vi "midterm_3.vi"() -> ()   [LabVIEW 2024]
uses:
  <userlib>/ME121-25-main/ME121-25-main/LabVIEW/SerialVIs/subs/portX.xctl
panel:
  in  "stop 3":bool
  out "Starting postion":cluster{"X":i32, "Y":i32}
  out "Ending Position":cluster{"X":i32, "Y":i32}
  out "2D Picture":picture
  in  "stop":bool
  in  "Initial Postion":cluster{"x-position":dbl, "y-position":dbl} {"y-position" scale=0.0..162.5; "x-position" scale=0.0..162.5}
  in  "Final Position":cluster{"x-position":dbl, "y-position":dbl} {"y-position" scale=0.0..162.5; "x-position" scale=0.0..162.5}
  out "Arms":picture
  in  "portX 2":refnum<visa-resource-name>(xcontrol)="ASRL15"
  in  "end effector":cluster{dbl, dbl}={159.01647214211073, 1.9100783062530127} {"?" format="%.1f"; "?" format="%#.1f"}
  in  "L 2":dbl(slide)=85.0 scale=0.0..200.0
  in  "L 1":dbl(slide)=77.5 scale=0.0..200.0
  out "resulting string":string="move(-43,72, -29)"
  # "Advance Dynamics - Midterm - 3DoF Arm"
  # "VI Overview\n\nThis LabVIEW VI controls a 3DoF robotic arm with two links and a chair attached to the end effector. \nThe objective is to move the arm while keeping the chair level to prevent a seated LEGO figure from falling.\nFeatures:\n\n    - Select initial and final positions\n    - Perform inverse kinematics (IK) to compute joint angles\n    - Communicate with a microcontroller to send movement commands\n    - Display a 2D visualization of the arm and its reachable workspace"
  # "1 - Select Port"
  # "User Guide:\n\n    1- Connect to the microcontroller via the port on the right.\n    2 -Select initial and final positions.\n    3 - Click Run:\n       - If the position is within range, a 2D visualization appears, and the user is prompted to execute the                                            \n          movement.\n       -  If out of range, the user is asked to select a valid position.\n\nLet me know if you need further refinements!"
  # "Set an initial position"
  # "mm"
  # "mm"
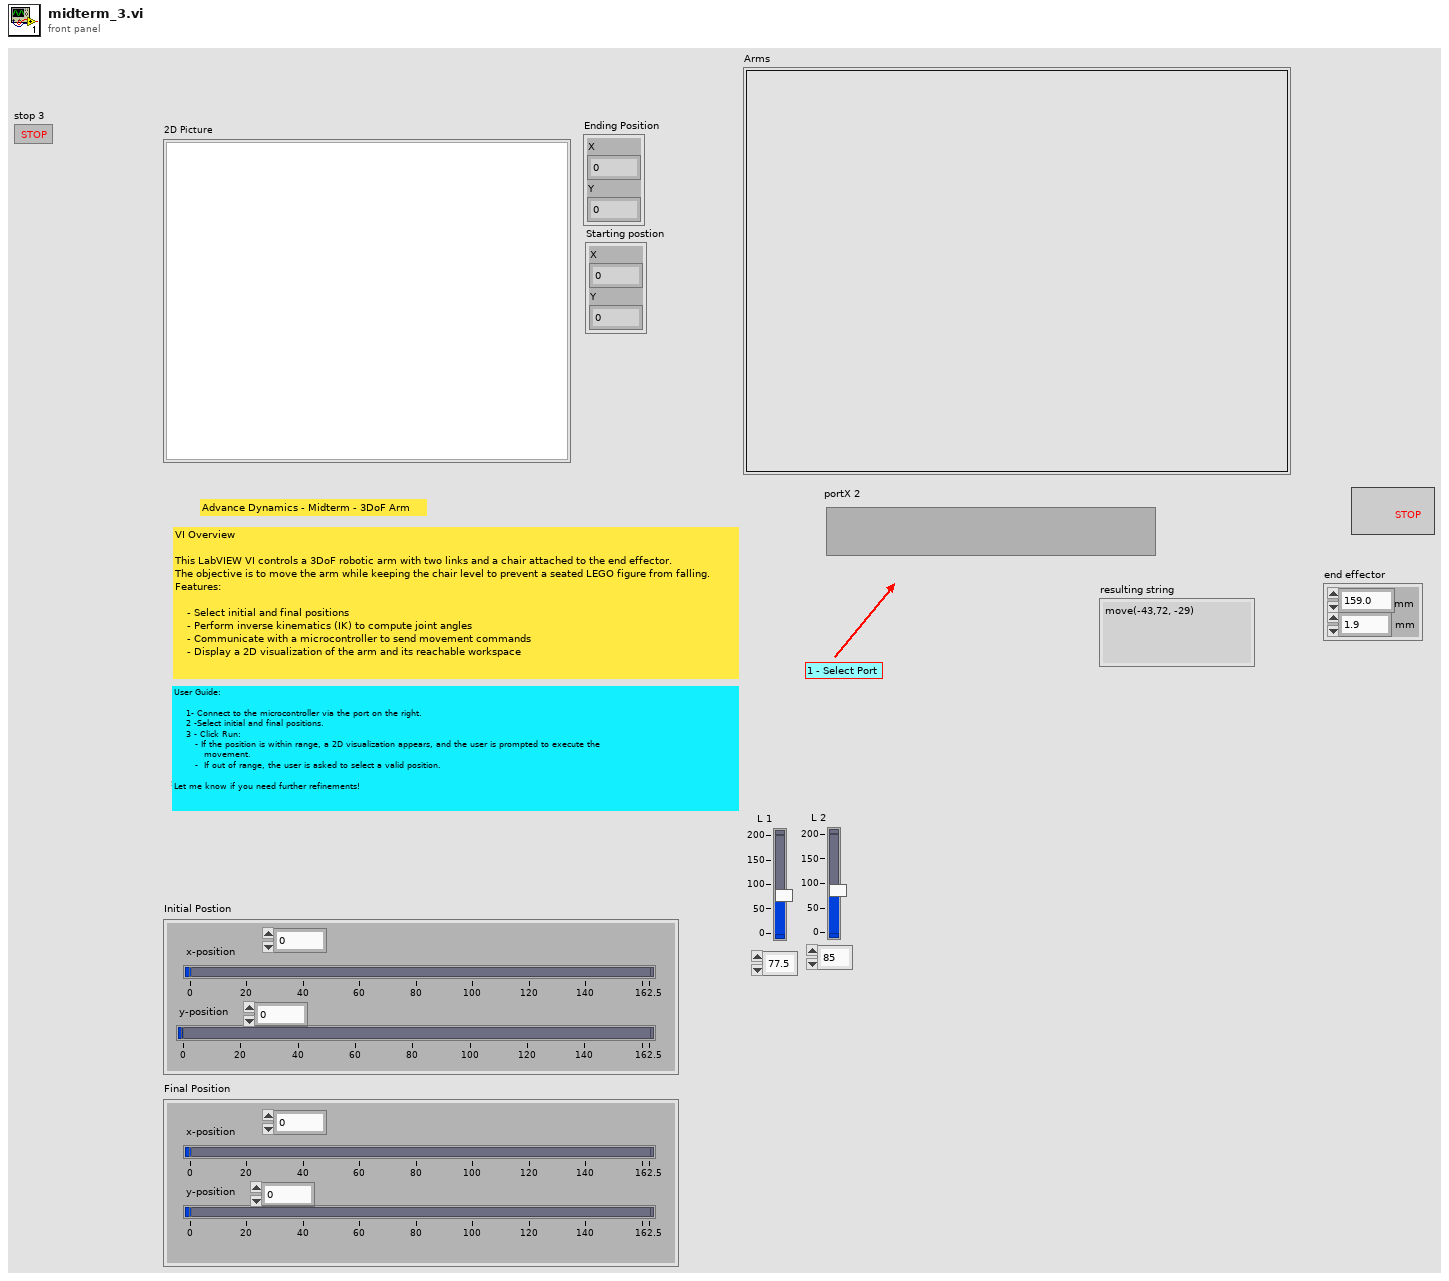
[diagram p1: front panel]
types:
  T1 = cluster{"Width":u16, "Style":enum32{"Solid", "Dash", "Dot", "DashDot", "DashDotDot"}}
  T2 = typedef "lveventtype.ctl" = enum32{"Null", "Timeout", "Annotation Menu Selection", "Annotation Menu Selection?", "App Instance Close", "App Instance Close?", "Autoscale Range Change", "Bookmark Info Change", "Cell Edit", "Cell Edit?", "Cursor Grab", "Cursor Grab?", "Cursor Menu Selection", "Cursor Menu Selection?", "Cursor Move", "Cursor Release", "Data Change", "Direction Change", "Display State Change", "Drag Ended", "Drag Enter", "Drag Leave", "Drag Over", "Drag Source Update", "Drag Starting", "Drag Starting?", "Drop", "Exec State Change", "Key Down", "Key Down?", "Key Repeat", "Key Repeat?", "Key Up", "Listbox Double Click", "Menu Activation?", "Menu Selection (App)", "Menu Selection? (App)", "Menu Selection (User)", "Mouse Down", "Mouse Down?", "Mouse Enter", "Mouse Leave", "Mouse Move", "Mouse Up", "Mouse Wheel", "NI Security User Change (App)", "Pane Size", "Panel Close", "Panel Close?", "Panel Resize", "Plot Attribute Change", "Scale Range Change", "Shortcut Menu Activation?", "Shortcut Menu Selection (App)", "Shortcut Menu Selection? (App)", "Shortcut Menu Selection (User)", "Tree Double Click", "Tree Drag", "Tree Drag?", "Tree Drop", "Tree Drop?", "Tree Item Close", "Tree Item Close?", "Tree Item Open", "Tree Item Open?", "User Event", "Value Change"}
  T3 = typedef "LVMouseTypeDef.ctl" = cluster{"Mouse Position":cluster{"X":i32, "Y":i32}, "Mouse Modifiers":cluster{"Button Down":bool, "Shift Mod":bool, "Menu Mod":bool, "Option Mod":bool}}
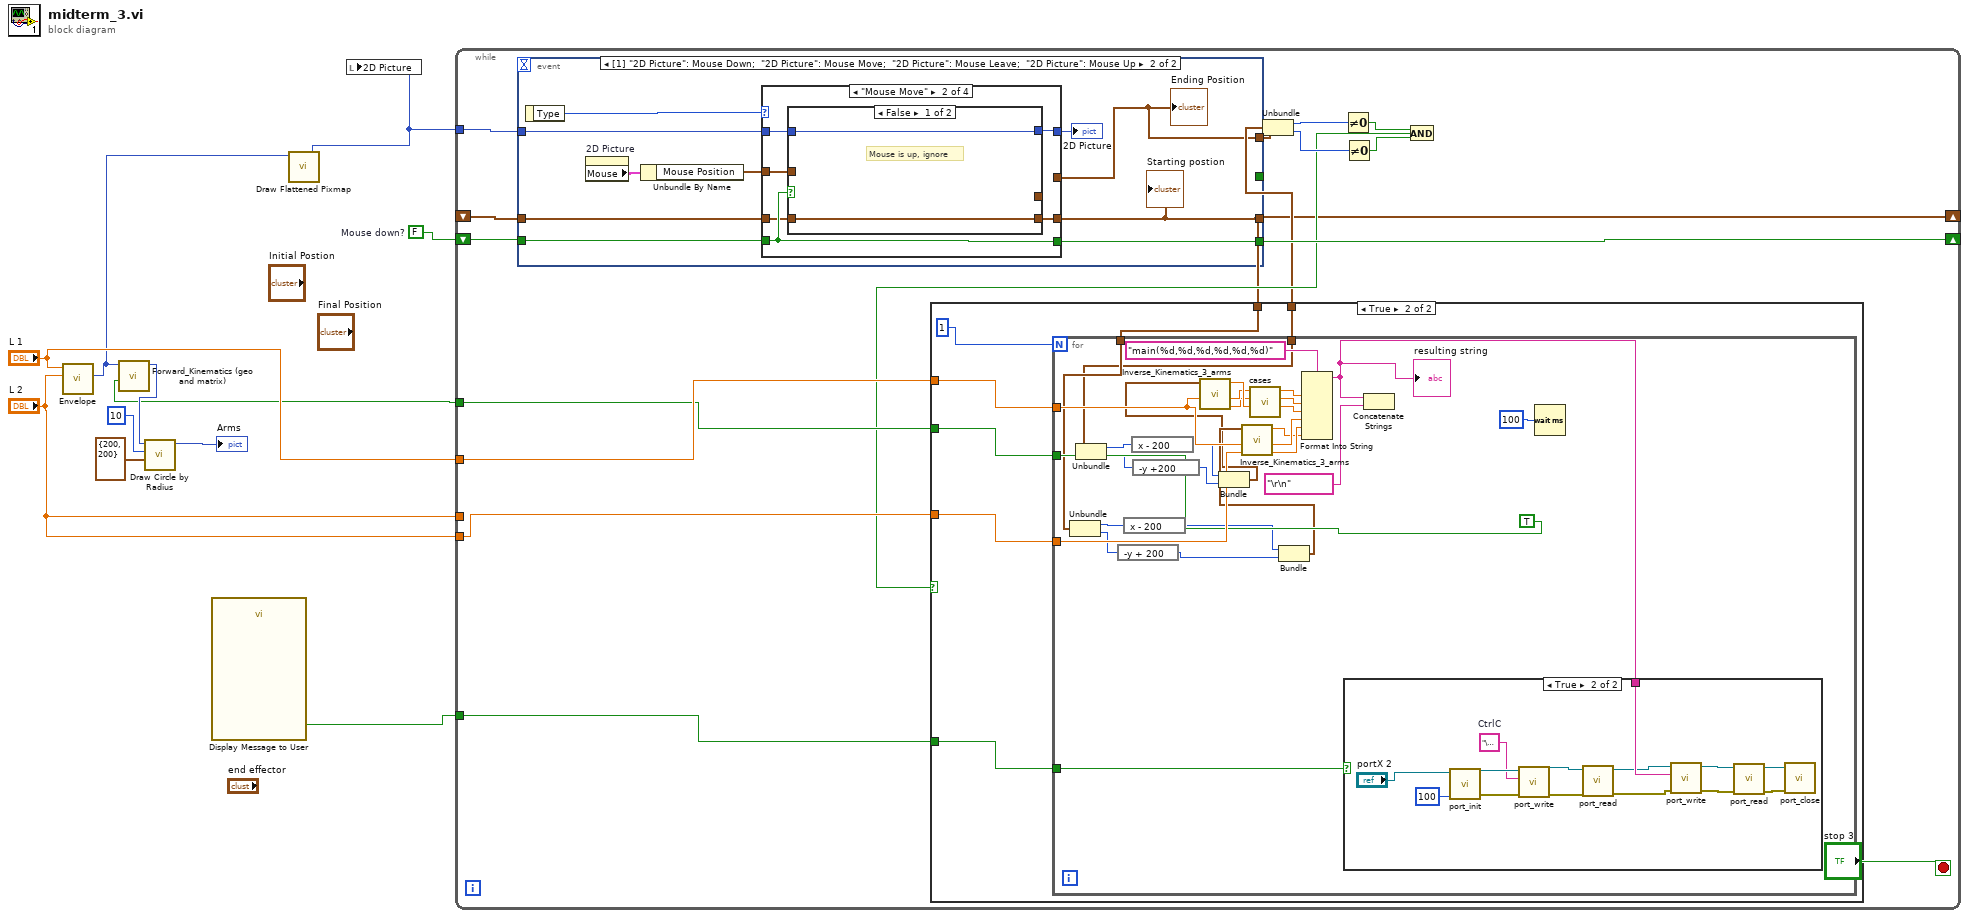
[diagram p0: block diagram]
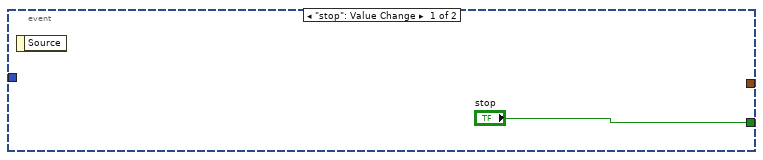
[diagram p4: hidden frame]
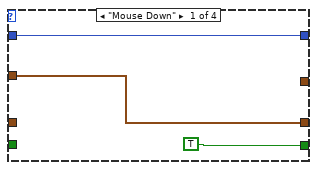
[diagram p5: hidden frame]
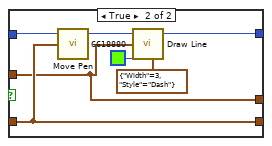
[diagram p6: hidden frame]
diagram:
  w10 = FALSE  # Mouse down?
  n1 = call "Envelope.vi"("L 2"="L 2", "L 1"="L 1") -> ("new picture"=w1:picture)  [unwired: 9 in]
  n2 = call "Display Message to User"() -> ("OK"=w2:bool)  [unwired: 10 in, 1 out]
  n3 = call <vilib>:"Draw Flattened Pixmap.vi"("picture"=w1) -> ("new picture"=w11:picture)  [unwired: 8 in]
  n4 = local write "2D Picture"(w11) -> ()
  n5 = while {
    tunnel: w11 -> [w27]
    shift-right: [w26] -> _
    shift-left: w10 -> [w25]
    shift-right: [w12] -> _
    shift-left: _ -> [w24]
    tunnel: "L 1" -> [w23]
    tunnel: "L 2" -> [_]
    tunnel: "L 2" -> [w22]
    tunnel: [w21] -> w3
    tunnel: w2 -> [w20]
    stop <- "stop 3" stop-if-true
    n6 = event shown="[1] \"2D Picture\": Mouse Down;  \"2D Picture\": Mouse Move;  \"2D Picture\": Mouse Leave;  \"2D Picture\": Mouse Up" {
      selector: _ -> [_ _]
      dyn-events: _ -> [_ _]
      timeout: _ -> [_ _]
      tunnel: ["stop" _] -> _
      tunnel: w27 -> [_ w86]
      tunnel: [_ w88] -> w26
      tunnel: w25 -> [_ w83]
      tunnel: [_ w82] -> w12
      tunnel: w24 -> [_ w81]
      tunnel: [_ w79] -> w13
      event "stop": Value Change {
        n7 = event-data() -> ()  [unwired: 1 in, 1 out]
      }
      event "2D Picture": Mouse Down; "2D Picture": Mouse Move; "2D Picture": Mouse Leave; "2D Picture": Mouse Up {
        n8 = event-data() -> ("Type"=w87:T2)  [unwired: 1 in]
        n9 = property on="2D Picture" class="Pict"() -> ("Mouse"=w84:T3)  [unwired: 2 in, 2 out]
        n10 = Unbundle By Name(w84) -> ("Mouse Position"=w80:cluster{"X":i32, "Y":i32})
        n11 = case shown="\"Mouse Move\"" w87 {
          tunnel: [TRUE ("fill?(F)") w94 _ _] -> w88
          tunnel: w86 -> [w89 w96 w108 w109]
          tunnel: [w89 w97 w108 w109] -> w85
          tunnel: w80 -> [w90 w95 _ w111]
          tunnel: w83 -> [_ w94 _ _]
          tunnel: [w90 w93 w107 w110] -> w82
          tunnel: w81 -> [_ w92 w107 w110]
          tunnel: [_ _ _ w111] -> w79
          frame "Mouse Down" {
          }
          frame "Mouse Move" {
            n12 = case shown="False" w94 {
              tunnel: [w99 w106] -> w97
              tunnel: w96 -> [w99 w104]
              tunnel: w95 -> [_ w100]
              tunnel: [w98 w102] -> w93
              tunnel: w92 -> [w98 w102]
              tunnel: [_ w100] -> _
              frame False {
                # "Mouse is up, ignore"
              }
              frame True {
                n13 = call <vilib>:"Move Pen.vi"("new position"=w102, "picture"=w104) -> ("new picture"=w103:picture)  [unwired: 3 in]
                n14 = call <vilib>:"Draw Line.vi"("picture"=w103, "end point"=w100, "color(black)"=u32 6618880, "pen"=T1 {"Width"=3, "Style"=enum."Dash"}) -> ("new picture"=w106:picture)  [unwired: 5 in]
              }
            }
          }
          frame Default {
            # "reset on mouse up, mouse leave, etc."
          }
          frame "Mouse Up" {
          }
        }
        "2D Picture" <- w85
        "Ending Position" <- w79
        "Starting postion" <- w82
      }
    }
    n15 = Unbundle(w13) -> ("X"=w18:i32, "Y"=w17:i32)
    n16 = Not Equal To 0?(x=w18) -> (x != 0?=w15:bool)
    n17 = Not Equal To 0?(x=w17) -> (x != 0?=w16:bool)
    n18 = And(x=w15, y=w16) -> (x .and. y?=w14:bool)
    n19 = case shown="True" w14 {
      tunnel: w23 -> [_ w33]
      tunnel: w22 -> [_ w32]
      tunnel: [_ w31] -> w21
      tunnel: w20 -> [_ w30]
      tunnel: w13 -> [_ w29]
      tunnel: w12 -> [_ w28]
      frame False {
      }
      frame True {
        n20 = for {
          N: 1 -> [_]
          tunnel: w33 -> [w60]
          tunnel: w32 -> [w59]
          tunnel: [TRUE ("geometry?")] -> w31
          tunnel: w30 -> [w47]
          tunnel: w29 -> [w43]
          tunnel: w28 -> [w46]
          n21 = Unbundle(w46) -> ("X"=w45:i32, "Y"=w44:i32)
          n22 = Unbundle(w43) -> ("X"=w42:i32, "Y"=w41:i32)
          n23 = expression code="-y + 200"(w44) -> (w39:i32)
          n24 = expression code="x - 200"(w45) -> (w40:i32)
          n25 = expression code="x - 200"(w42) -> (w37:i32)
          n26 = expression code="-y +200"(w41) -> (w36:i32)
          n27 = Bundle("X"=w37, "Y"=w36) -> (w35:cluster{"X":i32, "Y":i32})  [unwired: 1 in]
          n28 = call "Inverse_Kinematics_3_arms.vi"("L 1"=w60, "end effector"=w35) -> ("Angle 2"=w48:dbl, "Angle1"=w49:dbl, "Angle 3"=w50:dbl)  [unwired: 7 in]
          n29 = call "cases.vi"("q 3"=w50, "q 2"=w48, "q 1"=w49) -> ("q3"=w52:dbl, "q2"=w53:dbl, "q1"=w54:dbl)  [unwired: 6 in]
          n30 = Bundle("X"=w40, "Y"=w39) -> (w38:cluster{"X":i32, "Y":i32})  [unwired: 1 in]
          n31 = call "Inverse_Kinematics_3_arms.vi"("L 2"=w59, "L 1"=w60, "end effector"=w38) -> ("Angle 2"=w57:dbl, "Angle1"=w58:dbl, "Angle 3"=w56:dbl)  [unwired: 6 in]
          n32 = Format Into String(format string="main(%d,%d,%d,%d,%d,%d)", w54, w53, w52, w58, w57, w56) -> (resulting string=w55:string)  [unwired: 2 in, 1 out]
          "resulting string" <- w55
          n33 = case shown="True" w47 {
            tunnel: w55 -> [_ w75]
            frame False {
            }
            frame True {
              w68 = "\u0003"  # CtrlC
              n34 = call <userlib>:"port_init.vi"("Timeout (ms)"=u32 100, "VISA Refnum in"="portX 2") -> ("error out"=w73:errorcluster, "VISA Refnum out"=w74:refnum<visa-resource-name>)  [unwired: 8 in]
              n35 = call <userlib>:"port_write.vi"("error in (no error)"=w73, "write buffer"=w68, "VISA Refnum in"=w74) -> ("error out"=w71:errorcluster, "VISA Refnum out"=w72:refnum<visa-resource-name>)  [unwired: 7 in]
              n36 = call <userlib>:"port_read.vi"("error in (no error)"=w71, "VISA Refnum in"=w72) -> ("error out"=w67:errorcluster, "VISA Refnum out"=w66:refnum<visa-resource-name>)  [unwired: 7 in, 1 out]
              n37 = call <userlib>:"port_write.vi"("error in (no error)"=w67, "write buffer"=w75, "VISA Refnum in"=w66) -> ("error out"=w77:errorcluster, "VISA Refnum out"=w76:refnum<visa-resource-name>)  [unwired: 7 in]
              n38 = call <userlib>:"port_read.vi"("error in (no error)"=w77, "VISA Refnum in"=w76) -> ("error out"=w65:errorcluster, "VISA Refnum out"=w64:refnum<visa-resource-name>)  [unwired: 7 in, 1 out]
              n39 = call <userlib>:"port_close.vi"("error in (no error)"=w65, "VISA Refnum in"=w64) -> ()  [unwired: 10 in]
            }
          }
          n40 = Concatenate Strings(w55, "\r\n") -> ()  [unwired: 1 out]
          n41 = Wait (ms)(milliseconds to wait=u32 100) -> ()  [unwired: 1 out]
        }
      }
    }
  }
  n42 = call "Forward_Kinematics (geo and matrix).vi"("geometry?"=w3, "new picture"=w1) -> ("2D Picture"=w6:picture)  [unwired: 7 in, 2 out]
  n43 = call <vilib>:"Draw Circle by Radius.vi"("pixel center"=cluster{"horizontal":i16, "vertical":i16} {"horizontal"=200, "vertical"=200}, "radius"=i16 10, "picture"=w6) -> ("new picture"=→"Arms":picture)  [unwired: 8 in]
